vi "联合框控制选择结构.vi"() -> ()   [LabVIEW 2010]
panel:
  out "输出测试结果":string
  in  "选择测试内容":string(combo)
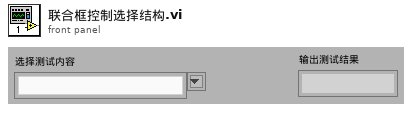
[diagram p1: front panel]
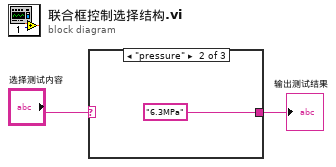
[diagram p0: block diagram]
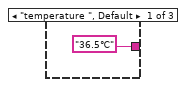
[diagram p2: hidden frame]
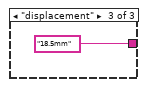
[diagram p3: hidden frame]
diagram:
  n1 = case shown="\"pressure\"" "选择测试内容" {
    tunnel: ["36.5℃" "6.3MPa" "18.5mm"] -> w1
    frame "temperature ", Default {
    }
    frame "pressure" {
    }
    frame "displacement" {
    }
  }
  "输出测试结果" <- w1
